vi "Recommed extenstion size.vi"(3 "size":u32) -> (1 "MsgPack Type":T1)   [LabVIEW 2020, in "MessagePack.lvlib" / "MsgPackExt.lvclass"]
uses:
  MsgPackExt.lvclass
  MsgPackExt.lvclass/MsgPackExt.ctl
  Typedefs/MsgPack Object Types.ctl
  MessagePack.lvlib
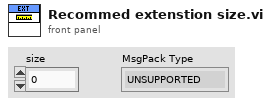
[diagram p1: front panel]
types:
  T1 = typedef "MessagePack.lvlib/MsgPack Object Types.ctl" = enum16{"UNSUPPORTED", "POSINT", "NEGINT", "FIXMAP", "FIXARRAY", "FIXSTR", "NIL", "FALSE", "TRUE", "BIN8", "BIN16", "BIN32", "EXT8", "EXT16", "EXT32", "FLOAT32", "FLOAT64", "UINT8", "UINT16", "UINT32", "UINT64", "INT8", "INT16", "INT32", "INT64", "FIXEXT1", "FIXEXT2", "FIXEXT4", "FIXEXT8", "FIXEXT16", "STR8", "STR16", "STR32", "ARRAY16", "ARRAY32", "MAP16", "MAP32"}
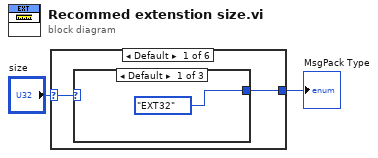
[diagram p0: block diagram]
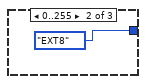
[diagram p2: hidden frame]
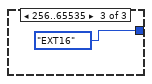
[diagram p3: hidden frame]
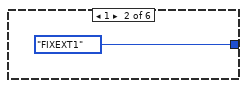
[diagram p4: hidden frame]
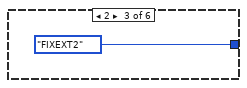
[diagram p5: hidden frame]
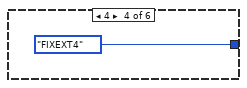
[diagram p6: hidden frame]
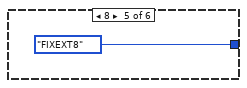
[diagram p7: hidden frame]
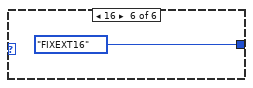
[diagram p8: hidden frame]
diagram:
  n1 = case shown="Default" "size" {
    selector: "size" -> [w4 _ _ _ _ _]
    tunnel: [w3 MsgPack_Object_Types."FIXEXT1" ("MsgPack Type") MsgPack_Object_Types."FIXEXT2" ("MsgPack Type") MsgPack_Object_Types."FIXEXT4" ("MsgPack Type") MsgPack_Object_Types."FIXEXT8" ("MsgPack Type") MsgPack_Object_Types."FIXEXT16" ("MsgPack Type")] -> w1
    frame Default {
      n2 = case shown="Default" w4 {
        tunnel: [MsgPack_Object_Types."EXT32" ("MsgPack Type") MsgPack_Object_Types."EXT8" ("MsgPack Type") MsgPack_Object_Types."EXT16" ("MsgPack Type")] -> w3
        frame Default {
        }
        frame 0..255 {
        }
        frame 256..65535 {
        }
      }
    }
    frame 1 {
    }
    frame 2 {
    }
    frame 4 {
    }
    frame 8 {
    }
    frame 16 {
    }
  }
  "MsgPack Type" <- w1
